vi "Measurement Logic.vi"() -> ()   [LabVIEW 2021, in "Generation_Class D Amplifier.lvlib"]
uses:
  Generation_Class D Amplifier.lvlib
  <vilib>/PDM Acquisition Toolkit/shared/controls/clock mode.ctl
  <vilib>/PDM Acquisition Toolkit/shared/PDM Shared.lvlib
  <vilib>/PDM Acquisition Toolkit/host/API/PDM Acquisition Toolkit.lvlib
  <vilib>/PDM Acquisition Toolkit/shared/controls/Digital Edge.ctl
  <vilib>/PDM Acquisition Toolkit/shared/controls/PCM Frame Sync Control.ctl
  <vilib>/PDM Acquisition Toolkit/shared/controls/PCM Data Justification.ctl
  <vilib>/PDM Acquisition Toolkit/shared/controls/PCM Bit Endianness.ctl
  <vilib>/PDM Acquisition Toolkit/shared/controls/PCM Data Format Configuration.ctl
  <vilib>/PDM Acquisition Toolkit/host/API/Public/Function Generator/Configure Custom Signal (N Ch) - PCM Output Task.vi
  Measurement Configuration.ctl
  Measurement Results.ctl
  shared/controls/units - snr.ctl
  shared/controls/audio controls.lvlib
  shared/controls/units - ratio.ctl
  <vilib>/MeasurementLink/MeasurementLink Measurement Server/Measure Call Context/Measure Call Context.lvclass
  shared/controls/digital audio protocol/data justification.ctl
  shared/controls/digital audio protocol/endianness.ctl
  shared/controls/digital audio protocol/digital edge.ctl
  shared/controls/weighting filter.ctl
  shared/controls/digital audio protocol/logic level.ctl
  shared/controls/digital output level units.ctl
  shared/controls/audio lowpass filter type.ctl
  shared/controls/audio highpass filter type.ctl
panel:
  out "Bit Clock Rate":sgl=3072000.0 format="%#_6pHz"
  out "measure call context out":refnum<class "Measure Call Context.lvclass">
  in  "measure call context in":refnum<class "Measure Call Context.lvclass">
  out "measurement results":T1={"channel names"=[], "frequency (Hz)"=[], "amplitude (Vrms)"=[], "amplitude (dBFS)"=[], "phase (deg)"=[], "SNR"=[], "THD+N"=[], "THD"=[], "dynamic range (dB)"=[], "gain"=[], "SFDR (dBc)"=[], "output power (W)"=[], "wfm - t0"=0.0, "wfm - dt"=1.9531249997269942e-05, "wfm - data"=array[12800 elements], "fft - f0"=0.0, "fft - df"=4.000000000559116, "fft - data"=array[6400 elements]}
  in  "measurement configuration":T2={"digital channel list"="7821\\PCMo 8", "frame clock rate"=48000.0, "number of channels"=2, "channel length"=32, "bit depth"=24, "data justification"=enum."Left Justified", "endianness"=enum."MSB First", "bit clock edge sync"=enum."Rising", "frame sync edge for channel 0"=enum."Rising", "channel 0 offset"=1, "master clock channel list"="7821\\PCMo 0", "master clock rate"=12288000.0, "enable dither"=FALSE, "logic level"=enum."3.3 V", "signal frequency"=1000.0, "output level"=1.0, "output level units"=enum."% FS", "output range (pk-pk)"=15.0, "load impedance"=4.0, "signal phase"=0.0, "acq sampling rate"=51200.0, "min measurement cycles"=20, "min measurement time (s)"=0.1, "min settling cycles"=0, "min settling time (s)"=0.005, "acq channel"="PXI1Slot4/ai0", "band start"=20.0, "band stop"=20000.0, "weighting filter"=enum."Linear", "lowpass filter"=enum."No filter", "highpass filter"=enum."DC", "SNR units"=enum."dB", "THD+N units"=enum."dB", "THD units"=enum."dB", "gain units"=enum."dB"} {"min settling cycles" format="%.3f"; "channel 0 offset" format="%#_6p"; "load impedance" format="%0.2f"; "acq sampling rate" format="%0.2f"; "frame clock rate" format="%#_6pHz"}
  out "error out":errorcluster
  in  "error in":errorcluster
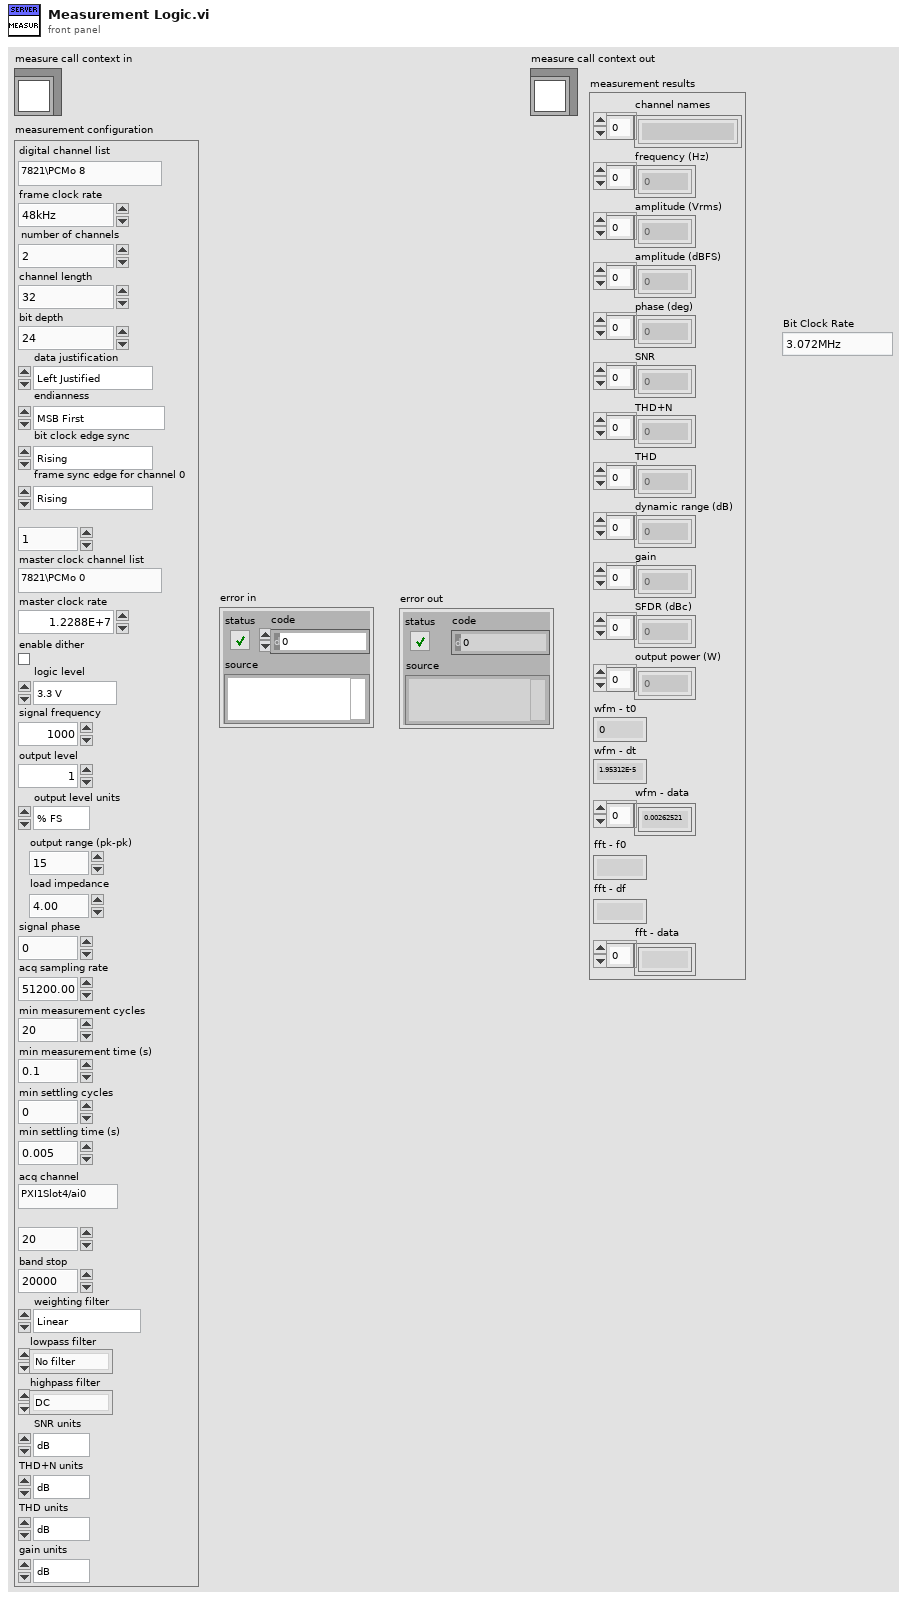
[diagram p1: front panel]
types:
  T1 = typedef "Generation_Class D Amplifier.lvlib/Measurement Results.ctl" = cluster{"channel names":string[], "frequency (Hz)":dbl[], "amplitude (Vrms)":dbl[], "amplitude (dBFS)":dbl[], "phase (deg)":dbl[], "SNR":dbl[], "THD+N":dbl[], "THD":dbl[], "dynamic range (dB)":dbl[], "gain":dbl[], "SFDR (dBc)":dbl[], "output power (W)":dbl[], "wfm - t0":dbl, "wfm - dt":dbl, "wfm - data":dbl[], "fft - f0":dbl, "fft - df":dbl, "fft - data":dbl[]}
  T2 = typedef "Generation_Class D Amplifier.lvlib/Measurement Configuration.ctl" = cluster{"digital channel list":string, "frame clock rate":dbl, "number of channels":u32, "channel length":u32, "bit depth":u32, "data justification":T3, "endianness":T4, "bit clock edge sync":T5, "frame sync edge for channel 0":T5, "channel 0 offset":u32, "master clock channel list":string, "master clock rate":dbl, "enable dither":bool, "logic level":T6, "signal frequency":dbl, "output level":dbl, "output level units":T7, "output range (pk-pk)":dbl, "load impedance":dbl, "signal phase":dbl, "acq sampling rate":dbl, "min measurement cycles":u32, "min measurement time (s)":dbl, "min settling cycles":u32, "min settling time (s)":dbl, "acq channel":string, "band start":dbl, "band stop":dbl, "weighting filter":T8, "lowpass filter":T9, "highpass filter":T10, "SNR units":T11, "THD+N units":T12, "THD units":T12, "gain units":T12}
  T3 = typedef "data justification.ctl" = enum32{"Left Justified", "Right Justified"}
  T4 = typedef "endianness.ctl" = enum32{"MSB First", "LSB First"}
  T5 = typedef "digital edge.ctl" = enum32{"Rising", "Falling"}
  T6 = typedef "logic level.ctl" = enum32{"3.3 V", "1.8 V", "1.2 V"}
  T7 = typedef "audio controls.lvlib/digital output level units.ctl" = enum32{"% FS", "dBFS"}
  T8 = typedef "weighting filter.ctl" = enum32{"Linear", "A-weighting", "B-weighting", "C-weighting"}
  T9 = typedef "audio controls.lvlib/audio lowpass filter type.ctl" = enum32{"No filter", "AES17 20kHz", "AES17 40kHz"}
  T10 = typedef "audio controls.lvlib/audio highpass filter type.ctl" = enum32{"DC", "AC"}
  T11 = typedef "audio controls.lvlib/units - snr.ctl" = enum32{"dB", "x/y"}
  T12 = typedef "audio controls.lvlib/units - ratio.ctl" = enum32{"dB", "%", "x/y"}
  T13 = typedef "PDM Shared.lvlib/PCM Data Format Configuration.ctl" = cluster{"Frame Sync Edge for Channel 0":T14, "Channel Count Per Frame":u8, "Channel Length":u16, "Bit Depth":u8, "Channel 0 Offset":u16, "Endianness":T15, "Data Justification":T16}
  T14 = typedef "PDM Shared.lvlib/Digital Edge.ctl" = enum8{"Rising", "Falling"}
  T15 = typedef "PDM Shared.lvlib/PCM Bit Endianness.ctl" = enum16{"MSB First", "LSB First"}
  T16 = typedef "PDM Shared.lvlib/PCM Data Justification.ctl" = enum16{"Left Justified", "Right Justified"}
  T17 = typedef "PDM Shared.lvlib/PCM Frame Sync Control.ctl" = cluster{"Frame Length":u16, "Frame Sync Pulse Width":u16, "Bit Clock Edge  Sync":T14}
  T18 = typedef "PDM Shared.lvlib/clock mode.ctl" = enum16{"divided clock", "DDS"}
  T19 = typedef "PDM Acquisition Class Library.lvlib/PCM Output Task.lvclass/PCM Output Task DVR.ctl" = refnum<data-value>
  T20 = typedef "PDM Acquisition Class Library.lvlib/I2S Output Task.lvclass/SignalProperties.ctl" = cluster{"cyclic signal":dbl[], "channel parameters":T21[]}
  T21 = typedef "PDM Acquisition Class Library.lvlib/I2S Output Channel.lvclass/GenerationChannelProperties.ctl" = cluster{"cyclic period":dbl, "cyclic phase offset":dbl, "gain":dbl}
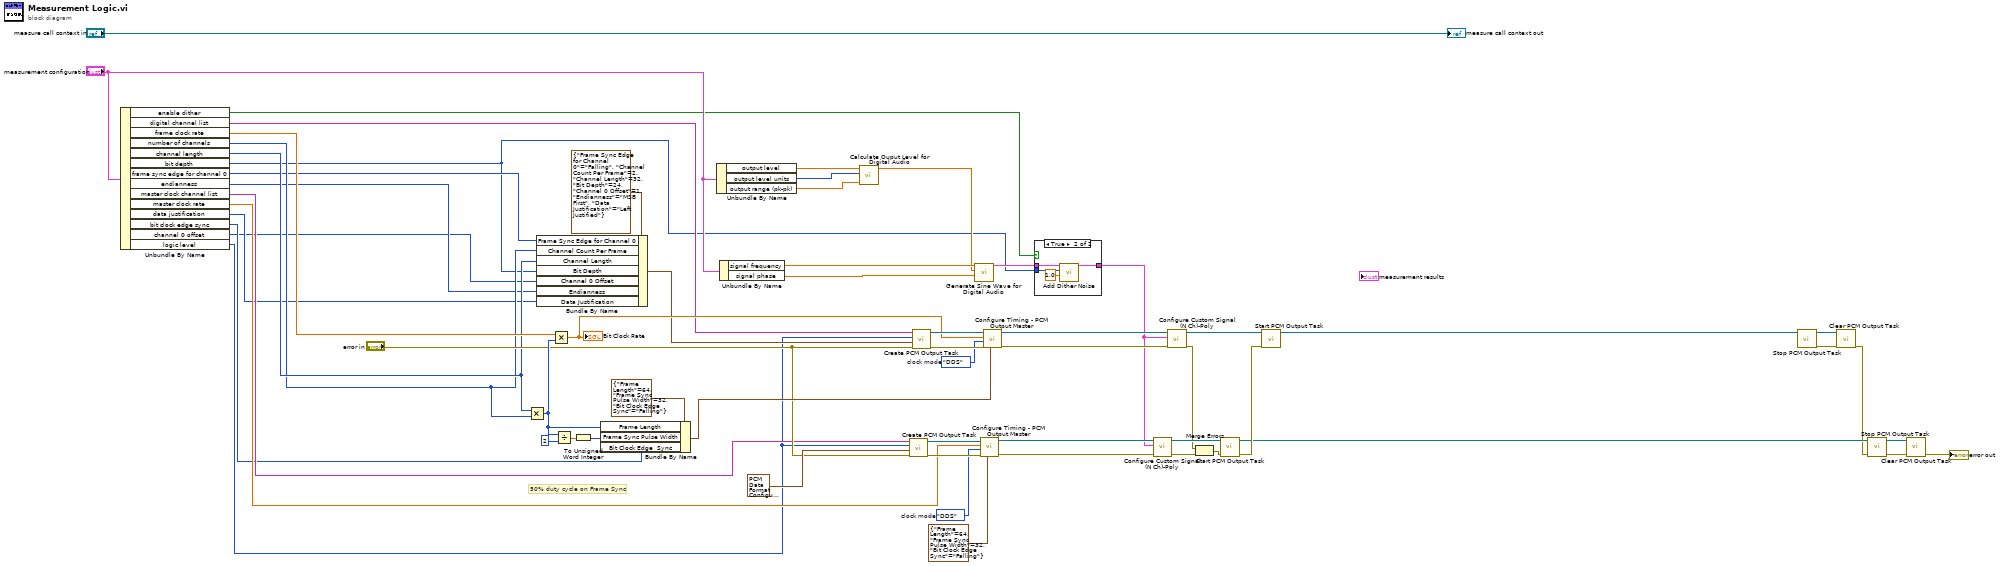
[diagram p0: block diagram]
diagram:
  w52 = clock_mode."DDS"  # clock mode
  w55 = clock_mode."DDS"  # clock mode
  # "50% duty cycle on Frame Sync"
  n1 = Unbundle By Name("measurement configuration") -> ("enable dither"=w1:bool, "digital channel list"=w6:string, "frame clock rate"=w25:dbl, "number of channels"=w23:u32, "channel length"=w24:u32, "bit depth"=w2:u32, "frame sync edge for channel 0"=w19:T5, "endianness"=w18:T4, "master clock channel list"=w22:string, "master clock rate"=w21:dbl, "data justification"=w20:T3, "bit clock edge sync"=w17:T5, "channel 0 offset"=w16:u32, "logic level"=w15:T6)
  n2 = Multiply(x=w24, y=w23) -> (x*y=w38:u32)
  n3 = Bundle By Name(cluster=T13 {"Frame Sync Edge for Channel 0"=enum."Falling", "Channel Count Per Frame"=2, "Channel Length"=32, "Bit Depth"=24, "Channel 0 Offset"=1, "Endianness"=enum."MSB First", "Data Justification"=enum."Left Justified"} ("PCM Data Configuration"), "Frame Sync Edge for Channel 0"=w19, "Channel Count Per Frame"=w23, "Channel Length"=w24, "Bit Depth"=w2, "Channel 0 Offset"=w16, "Endianness"=w18, "Data Justification"=w20) -> (w35:T13)
  n4 = Multiply(x=w25, y=w38) -> (x*y=w37:dbl)
  "Bit Clock Rate" <- w37
  n5 = Divide(x=w38, y=u16 2) -> (x/y=w40:dbl)
  n6 = To Unsigned Word Integer(number=w40) -> (unsigned 16bit integer=w39:u16)
  n7 = Bundle By Name(cluster=T17 {"Frame Length"=64, "Frame Sync Pulse Width"=32, "Bit Clock Edge  Sync"=enum."Falling"} ("Frame Sync Clock Control"), "Frame Length"=w38, "Frame Sync Pulse Width"=w39, "Bit Clock Edge  Sync"=w17) -> (w42:T17)
  n8 = Unbundle By Name("measurement configuration") -> ("output level"=w9:dbl, "output level units"=w8:T7, "output range (pk-pk)"=w7:dbl)
  n9 = Unbundle By Name("measurement configuration") -> ("signal frequency"=w13:dbl, "signal phase"=w14:dbl)
  n10 = call "Calculate Ouput Level for Digital Audio.vi"("output range (pk-pk)"=w7, "digital output level units"=w8, "output level"=w9) -> ("gain"=w12:dbl)  [unwired: 7 in, 1 out]
  n11 = call <vilib>:"Create PCM Output Task.vi"("error in"="error in", "PCM data configuration"=T13 {"Frame Sync Edge for Channel 0"=enum."Falling", "Channel Count Per Frame"=2, "Channel Length"=32, "Bit Depth"=24, "Channel 0 Offset"=1, "Endianness"=enum."MSB First", "Data Justification"=enum."Left Justified"} ("PCM Data Configuration 2"), "logic level"=w15, "channel list"=w22) -> ("error out"=w53:errorcluster, "PCM output task out"=w54:T19)  [unwired: 6 in]
  n12 = call <vilib>:"Create PCM Output Task.vi"("error in"="error in", "PCM data configuration"=w35, "logic level"=w15, "channel list"=w6) -> ("error out"=w56:errorcluster, "PCM output task out"=w57:T19)  [unwired: 6 in]
  n13 = call "Generate Sine Wave for Digital Audio.vi"("phase"=w14, "gain"=w12, "frequency"=w13) -> ("Signal Properties"=w4:T20)  [unwired: 8 in]
  n14 = call <vilib>:"Configure Timing - PCM Output Master.vi"("Frame Sync Clock Control"=T17 {"Frame Length"=64, "Frame Sync Pulse Width"=32, "Bit Clock Edge  Sync"=enum."Falling"} ("Frame Sync Clock Control 2"), "error in"=w53, "clock mode"=w52, "Bit Clock rate"=w21, "PCM output task in"=w54) -> ("error out"=w34:errorcluster, "PCM output task out"=w33:T19)  [unwired: 4 in, 1 out]
  n15 = call <vilib>:"Configure Timing - PCM Output Master.vi"("Frame Sync Clock Control"=w42, "error in"=w56, "clock mode"=w55, "Bit Clock rate"=w37, "PCM output task in"=w57) -> ("error out"=w10:errorcluster, "PCM output task out"=w11:T19)  [unwired: 4 in, 1 out]
  n16 = case shown="True" w1 {
    tunnel: w4 -> [w61 w65]
    tunnel: [w61 w64] -> w3
    tunnel: w2 -> [_ w63]
    frame False {
    }
    frame True {
      n17 = call "Add Dither Noise.vi"("amplitude (LSB)"=1.0, "bits"=w63, "Signal Properties"=w65) -> ("Signal Properties"=w64:T20)  [unwired: 8 in]
    }
  }
  n18 = call-poly <vilib>:"Configure Custom Signal (N Ch)-Poly.vi"("error in"=w34, "signal parameters"=w3, "PCM output task in"=w33) -> ("error out"=w29:errorcluster, "PCM output task out"=w32:T19)  [unwired: 7 in]
  n19 = call-poly <vilib>:"Configure Custom Signal (N Ch)-Poly.vi"("error in"=w10, "signal parameters"=w3, "PCM output task in"=w11) -> ("error out"=w30:errorcluster, "PCM output task out"=w31:T19)  [unwired: 7 in]
  n20 = Merge Errors(w30, w29) -> (w48:errorcluster)
  n21 = call <vilib>:"Start PCM Output Task.vi"("error in"=w48, "PCM output task in"=w32) -> ("error out"=w49:errorcluster, "PCM output task out"=w45:T19)  [unwired: 8 in]
  n22 = call <vilib>:"Start PCM Output Task.vi"("error in"=w49, "PCM output task in"=w31) -> ("PCM output task out"=w28:T19)  [unwired: 8 in, 1 out]
  n23 = call <vilib>:"Stop PCM Output Task.vi"("PCM output task In"=w28) -> ("error out"=w59:errorcluster, "PCM output task out"=w58:T19)  [unwired: 9 in]
  n24 = call <vilib>:"Clear PCM Output Task.vi"("error in"=w59, "PCM output task in"=w58) -> ("error out"=w44:errorcluster)  [unwired: 9 in]
  n25 = call <vilib>:"Stop PCM Output Task.vi"("error in"=w44, "PCM output task In"=w45) -> ("error out"=w47:errorcluster, "PCM output task out"=w46:T19)  [unwired: 8 in]
  n26 = call <vilib>:"Clear PCM Output Task.vi"("error in"=w47, "PCM output task in"=w46) -> ("error out"=→"error out":errorcluster)  [unwired: 9 in]
  "measure call context out" <- "measure call context in"
